vi "SendToAll.vi"(6 "Priority Message? (F)":bool, 8 "error in (no error)":errorcluster, 9 "Data":variant, 10 "Message":string, 11 "Message Queues":T1) -> (0 "error out":errorcluster)   [LabVIEW 2017, in "Client.lvlib" / "CommsFrameWork.lvlib"]
doc: "Sends a Message to all Message-Queues except the MHL. This is used for broadcasting Initialize and Exit Messages (and maybe others that every loop needs)."
uses:
  CommsFrameWork.lvlib
  TypeDefs/CommReferences.ctl
  TypeDefs/MessageCluster.ctl
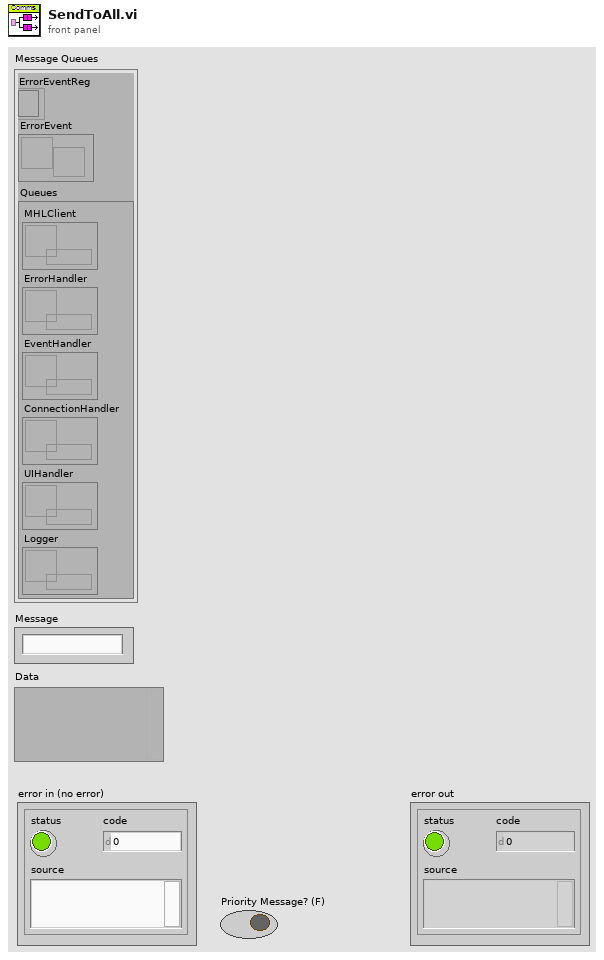
[diagram p1: front panel]
types:
  T1 = typedef "Client.lvlib/CommsFrameWork.lvlib/CommReferences.ctl" = cluster{"ErrorEventReg":refnum<event-registration>, "ErrorEvent":refnum<user-event>, "Queues":cluster{"MHLClient":refnum<queue>, "ErrorHandler":refnum<queue>, "EventHandler":refnum<queue>, "ConnectionHandler":refnum<queue>, "UIHandler":refnum<queue>, "Logger":refnum<queue>}}
  T2 = cluster{"MHLClient":refnum<queue>, "ErrorHandler":refnum<queue>, "EventHandler":refnum<queue>, "ConnectionHandler":refnum<queue>, "UIHandler":refnum<queue>, "Logger":refnum<queue>}
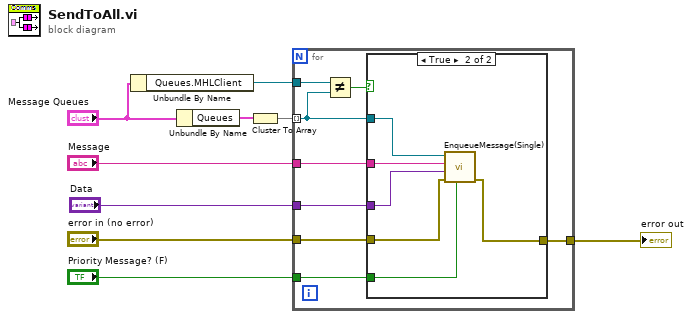
[diagram p0: block diagram]
diagram:
  n1 = Unbundle By Name("Message Queues") -> ("Queues.MHLClient"=w3:refnum<queue>)
  n2 = Unbundle By Name("Message Queues") -> ("Queues"=w1:T2)
  n3 = Cluster To Array(cluster=w1) -> (array=w9:refnum<queue>[])
  n4 = for {
    tunnel: w9 -> [w11] mode=indexing
    tunnel: "Message" -> [w17]
    tunnel: "Data" -> [w16]
    tunnel: "error in (no error)" -> [w15]
    tunnel: "Priority Message? (F)" -> [w14]
    tunnel: [w13] -> w4
    tunnel: w3 -> [w12]
    n5 = Not Equal?(x=w12, y=w11) -> (x != y?=w10:bool)
    n6 = case shown="True" w10 {
      tunnel: w17 -> [_ w24]
      tunnel: w16 -> [_ w23]
      tunnel: w15 -> [w18 w22]
      tunnel: w14 -> [_ w21]
      tunnel: [w18 w20] -> w13
      tunnel: w11 -> [_ w19]
      frame False {
      }
      frame True {
        n7 = call "EnqueueMessage(Single).vi"("Priority Message? (F)"=w21, "error in (no error)"=w22, "Message Data"=w23, "Message"=w24, "Message Queue"=w19) -> ("error out"=w20:errorcluster)  [unwired: 5 in, 1 out]
      }
    }
  }
  "error out" <- w4
